vi "SIM_CurrentOutput.vi"(9 "array":dbl[][](array[numeric]), 10 "y":dbl, 11 "x":dbl) -> (2 "Zread":dbl)   [LabVIEW 2019]
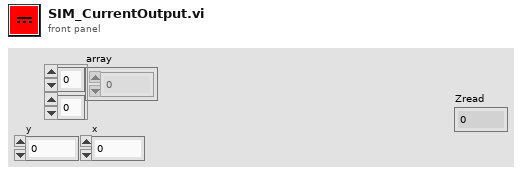
[diagram p1: front panel]
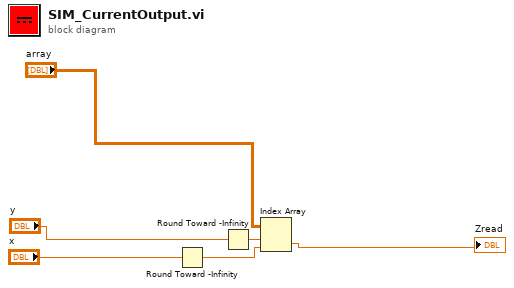
[diagram p0: block diagram]
diagram:
  n1 = Round Toward -Infinity(1:"x") -> (0:w5:dbl)
  n2 = Round Toward -Infinity(1:"y") -> (0:w6:dbl)
  n3 = Index Array(array="array", index (row)=w6, index (col)=w5) -> (element=→"Zread":dbl)
